vi "Read Request URI.vi"(8 "error in (no error)":errorcluster, 11 "ErrorOrSuccess in":refnum<class "ErrorOrSuccess.lvclass">) -> (0 "error out":errorcluster, 2 "Request URI":string, 3 "ErrorOrSuccess out":refnum<class "ErrorOrSuccess.lvclass">)   [LabVIEW 2020, in "wamplv.lvlib" / "ErrorOrSuccess.lvclass"]
uses:
  ErrorOrSuccess.lvclass
  ErrorOrSuccess.lvclass/ErrorOrSuccess.ctl
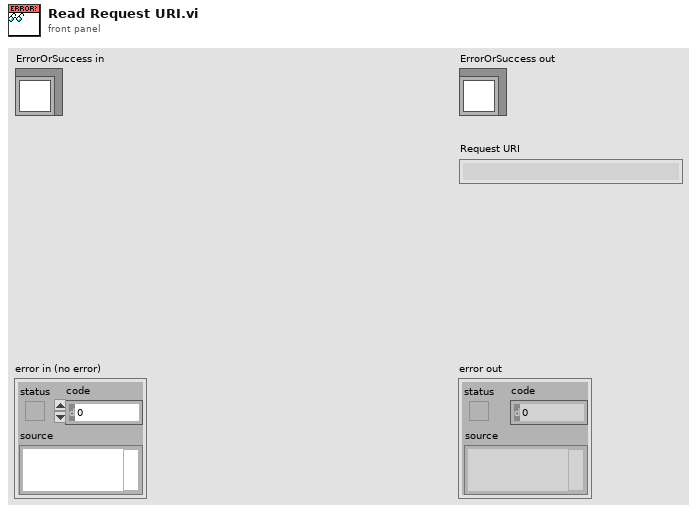
[diagram p1: front panel]
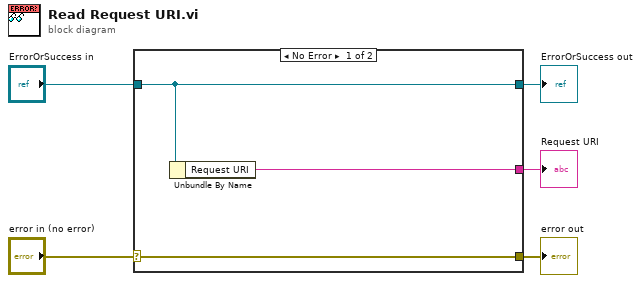
[diagram p0: block diagram]
diagram:
  n1 = case shown="No Error" "error in (no error)" {
    selector: "error in (no error)" -> [w8 w9]
    tunnel: [w8 w9] -> w4
    tunnel: [w7 w10] -> w2
    tunnel: "ErrorOrSuccess in" -> [w7 w10]
    tunnel: [w6 _] -> w1
    frame No Error {
      n2 = Unbundle By Name(w7) -> ("Request URI"=w6:string)
    }
    frame Error {
    }
  }
  "error out" <- w4
  "ErrorOrSuccess out" <- w2
  "Request URI" <- w1
